vi "Encode.vi"(8 "error in (no error)":errorcluster, 11 "Felica DOWN in":refnum<class "Felica DOWN.lvclass">) -> (0 "error out":errorcluster, 3 "Felica DOWN out":refnum<class "Felica DOWN.lvclass">)   [LabVIEW 2019, in "Felica DOWN.lvclass"]
uses:
  Felica DOWN.lvclass
  TypeDef/Store.ctl
  Felica DOWN.lvclass/Felica DOWN.ctl
  RFID system.lvclass
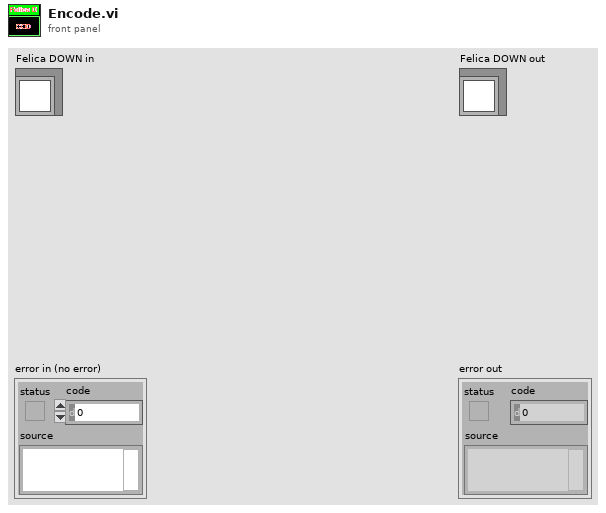
[diagram p1: front panel]
types:
  T1 = typedef "Store.ctl" = enum16{"envelope", "noise", "demSubCar", "CH_frame", "Decode", "demodulate", "in", "out", "sum", "subCarrier", "frame", "command", "encode", "modulate", "encode_UP", "modulate_up", "demod_up", "envelop_up", "sum_up", "out_up", "in_up"}
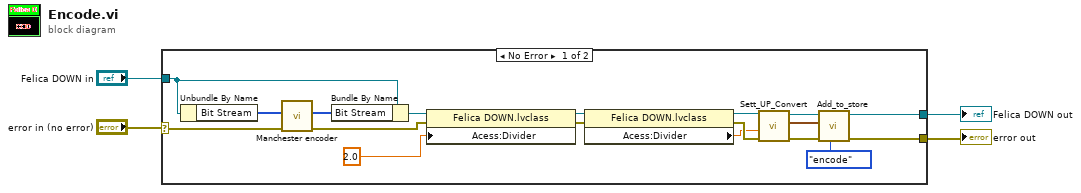
[diagram p0: block diagram]
diagram:
  n1 = case shown="No Error" "error in (no error)" {
    selector: "error in (no error)" -> [w21 w23]
    tunnel: [w14 w23] -> w3
    tunnel: "Felica DOWN in" -> [w20 w24]
    tunnel: [w16 w24] -> w1
    frame No Error {
      n2 = Unbundle By Name(w20) -> ("Bit Stream"=w22:u8[])
      n3 = call "Manchester encoder.vi"("Error In"=w21, "Bit stream in"=w22) -> ("error out"=w10:errorcluster, "Bit stream out (Manchester encode)"=w19:u8[])  [unwired: 8 in]
      n4 = Bundle By Name(cluster=w20, "Bit Stream"=w19) -> (w18:refnum<class "Felica DOWN.lvclass">)
      n5 = property class="Felica DOWN.lvclass"(reference=w18, error in=w10, "Acess:Divider"=2.0 ("Divider")) -> (reference out=w11:refnum<class "Felica DOWN.lvclass">, error out=w7:errorcluster)
      n6 = property class="Felica DOWN.lvclass"(reference=w11, error in=w7) -> (reference out=w8:refnum<class "Felica DOWN.lvclass">, error out=w6:errorcluster, "Acess:Divider"=w5:dbl)
      n7 = call-dynamic "Sett_UP_Convert.vi"("error in (no error)"=w6, "Divider(1)"=w5, "Felica DOWN in"=w8) -> ("error out"=w15:errorcluster, "Waveform"=w13:waveform(dbl), "Felica DOWN out"=w17:refnum<class "Felica DOWN.lvclass">)  [unwired: 6 in]
      n8 = call "Add_to_store.vi"("Store"=Store."encode", "error in (no error)"=w15, "Waveform"=w13, "RFID system in"=w17) -> ("error out"=w14:errorcluster, "RFID system out"=w16:refnum<class "Felica DOWN.lvclass">)  [unwired: 6 in]
    }
    frame Error {
    }
  }
  "error out" <- w3
  "Felica DOWN out" <- w1
